vi "Review_Scan_Data.vi"(8 "error in (no error)":errorcluster) -> (0 "error out":errorcluster)   [LabVIEW 2017]
uses:
  Q Driver/Controls/Review_Q options.ctl
  Q Driver/Controls/Review EnQ.ctl
  Controls/Main Cluster.ctl
  Controls/GUI Reference Cluster.ctl
  SQL/SQL/SQL_DB-Enum.ctl
  SQL/Detailed Report _Colums_Informatin.ctl
  <vilib>/addons/database/Auxilliary.llb/DB Tools DataTypes.ctl
  DB Driver/DB Driver Main Options.ctl
  <vilib>/addons/database/NI_Database_API.lvlib
panel:
  out "Machine Tested TIME":dbl(knob) scale=0.0..3000.0
  in  "Search Type":string(combo)="Date&Time"
  out "TESTED":dbl(slide) scale=0.0..10.0
  out "FAIL":dbl(slide) scale=0.0..10.0
  out "PASS":dbl(slide) scale=0.0..10.0
  in  "Table":i32(listbox)=-1
  in  "Password":string caption="User_Name"
  in  "User ID":string caption="User_Name"
  out "DB Name":string
  out "DB Connection Status":string
  out "User Instruction":string
  in  "Export to Pdf":bool
  in  "Close":bool
  in  "Export to CSV":bool
  in  "All/ Top 1000":bool
  in  "Select Field":string(combo)
  in  "Tables":string(combo)
  in  "Field Data":string
  in  "To Date":timestamp
  in  "From Date":timestamp
  in  "Search Data":bool
  out "Connection":bool
  in  "Connect":bool
  out "SERVER NAME :":string
  out "date/time string":string="Wednesday, November 13 2013 2:41:59 PM"
  # "Data Base Connection"
  # "User ID"
  # "Password"
  # "Report Viewer"
  # "Search And Export"
  # "To Date"
  # "From Date"
  # "S.No"
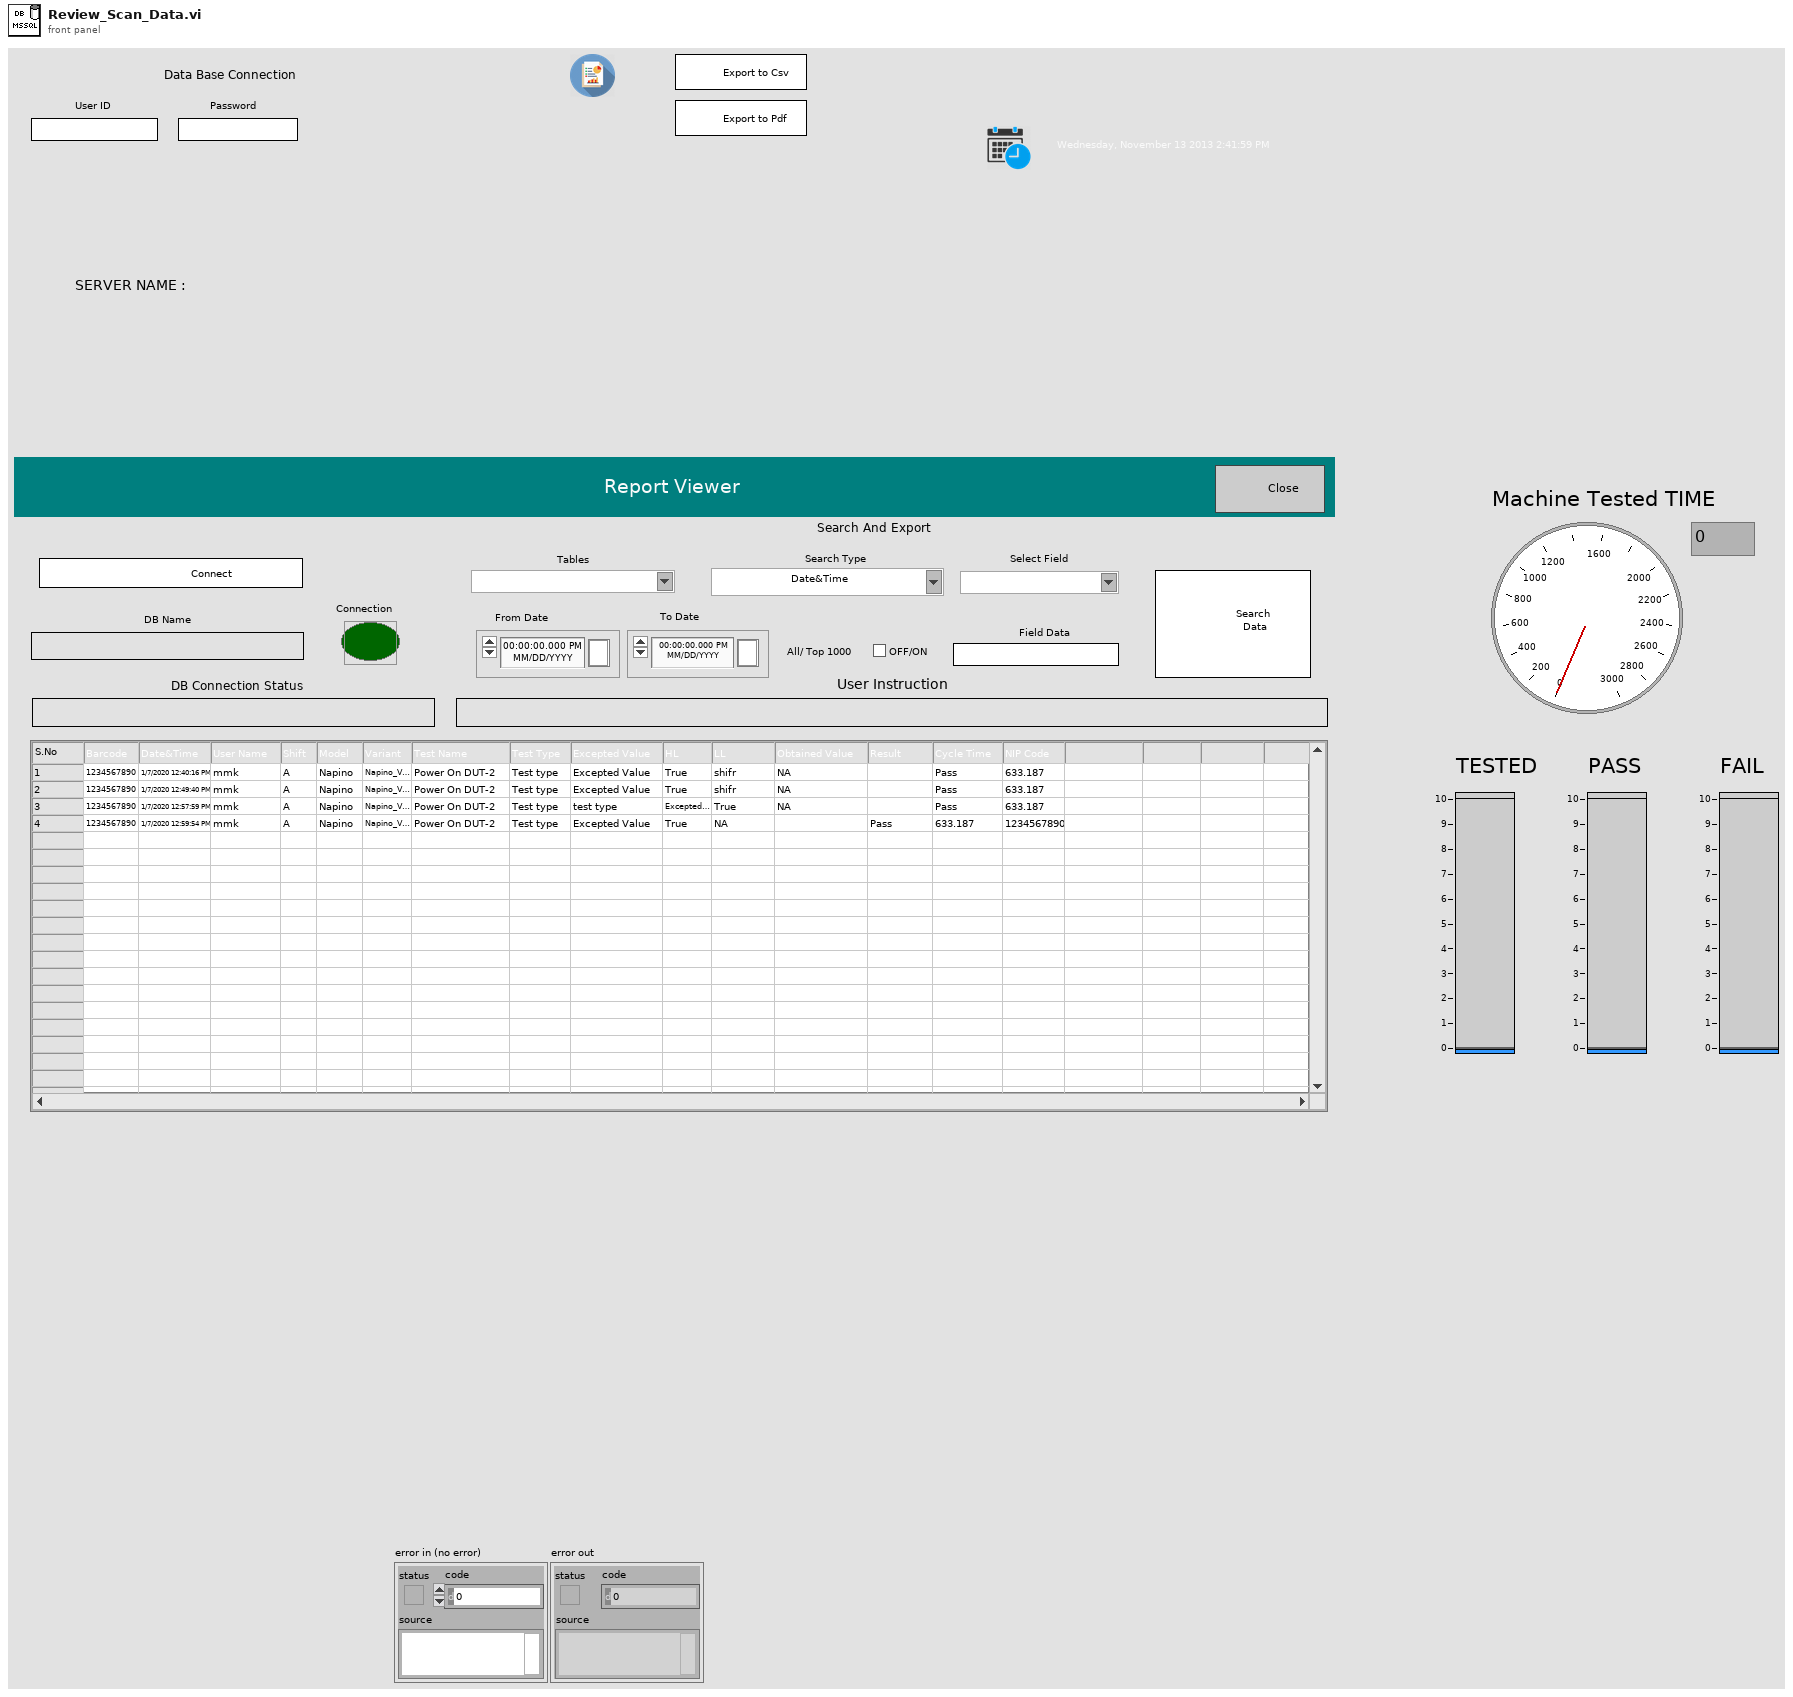
[diagram p1: front panel]
types:
  T1 = typedef "Main Cluster.ctl" = cluster{"From Date":timestamp, "To Date":timestamp, "Selected Database":string, "Selected Table":string, "Selected Field":string, "Field Data":string, "DB Connection Ststus":string, "User Instruction":string, "All/ Top 1000":bool, "Table Data":string[][], "Query":string, "Selected Server":string, "Connection Status":bool, "User ID":string, "Password":string, "Date/Field":bool, "(Date/Field/All)":enum8{"False", "True", "Mixed"}, "First Run":bool, "Selected DB Tables":string[], "From Date Field":string, "To Date Field":string, "Selected Table Fields":string[], "Search Type":string, "Reference":T2, "Mahine RUN Time":dbl, "Pass/Fail querry":string}
  T2 = typedef "GUI Reference Cluster.ctl" = cluster{"Top 1000/ All":refnum<vi>, "Search by date":refnum<vi>, "From Date":refnum<vi>, "Select Field":refnum<vi>, "Field Data":refnum<vi>, "To Date":refnum<vi>, "Tables":refnum<vi>, "Search Type":refnum<vi>}
  T3 = typedef "Review EnQ.ctl" = enum16{"Poll", "Init", "Connect", "Close", "Generate Query", "Update", "Take All Reference", "Check Tables & Create", "Read DB", "Export to Pdf", "Export to Csv", "Error", "Exit"}
  T4 = typedef "Review_Q options.ctl" = enum16{"Init", "En Q", "EN Q N", "EN Q Stack", "EN Q Stack N", "De Q", "Flush", "Close"}
  T5 = typedef "SQL_DB-Enum.ctl" = enum16{"INI DATA", "Open Connections", "Query", "Update Table", "Get Full Report", "Get Serial Numbers", "Get Table Columns", "Get Table Names", "Check & Create Table", "Close Connection"}
  T6 = typedef "Detailed Report _Colums_Informatin.ctl" = cluster{"column name":string, "data type":T7, "size":i32, "allow null?":bool}[]
  T7 = typedef "NI_Database_API.lvlib/DB Tools DataTypes.ctl" = enum16{"String", "Long (I32)", "Single (SGL)", "Double (DBL)", "Date/Time", "Binary"}
  T8 = typedef "DB Driver Main Options.ctl" = enum16{"Open", "RefOut", "Select", "Execute", "Update", "Insert 2D", "Insert OrUpdate", "Close"}
  T9 = cluster{"left":i16, "top":i16, "right":i16, "bottom":i16}
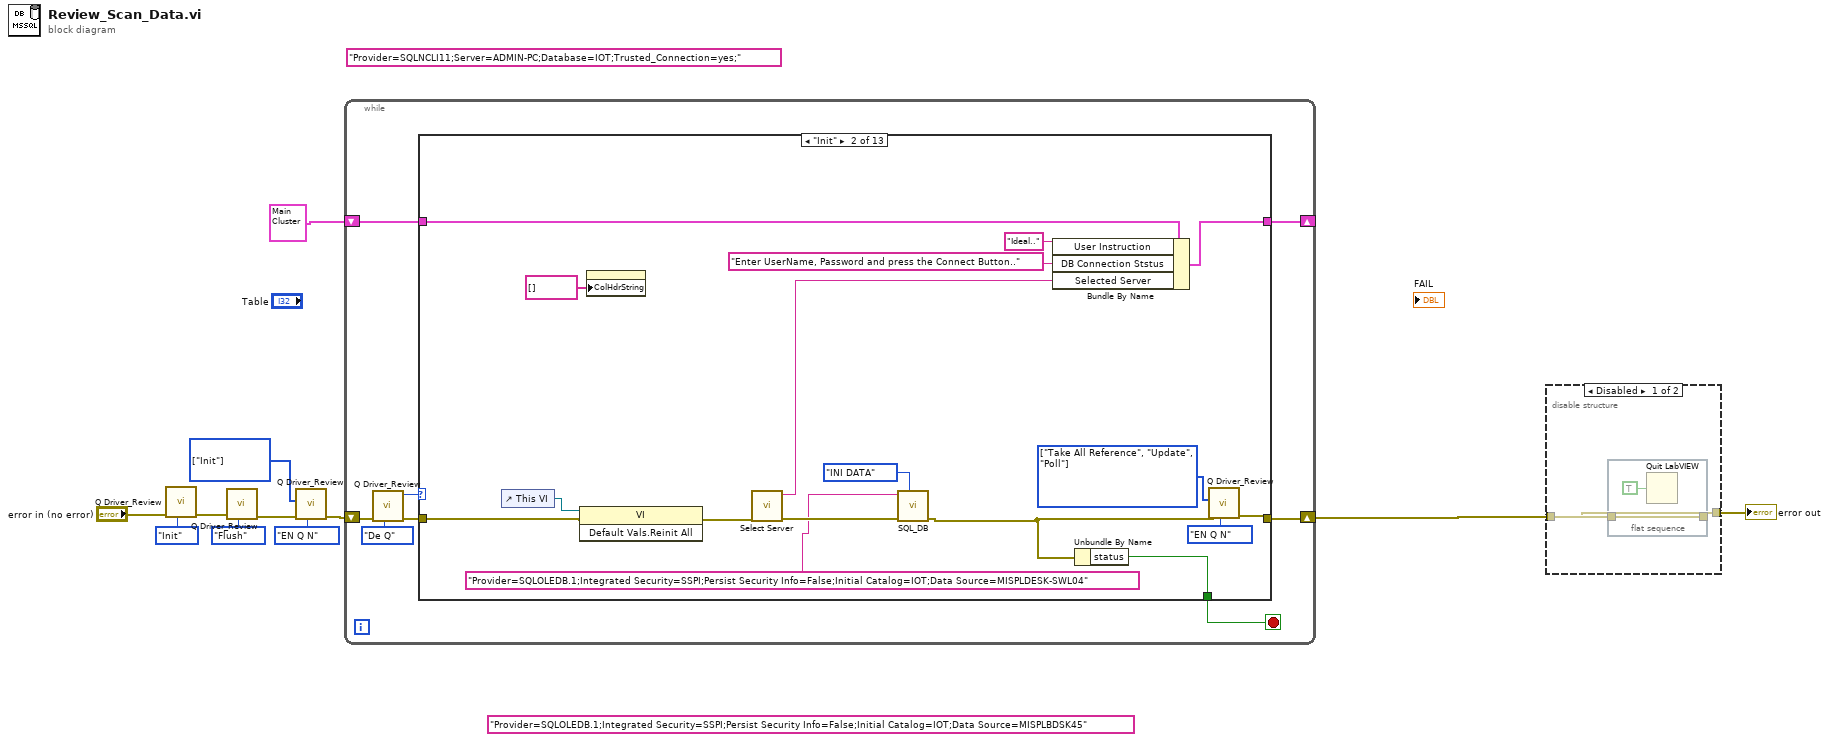
[diagram p0: block diagram]
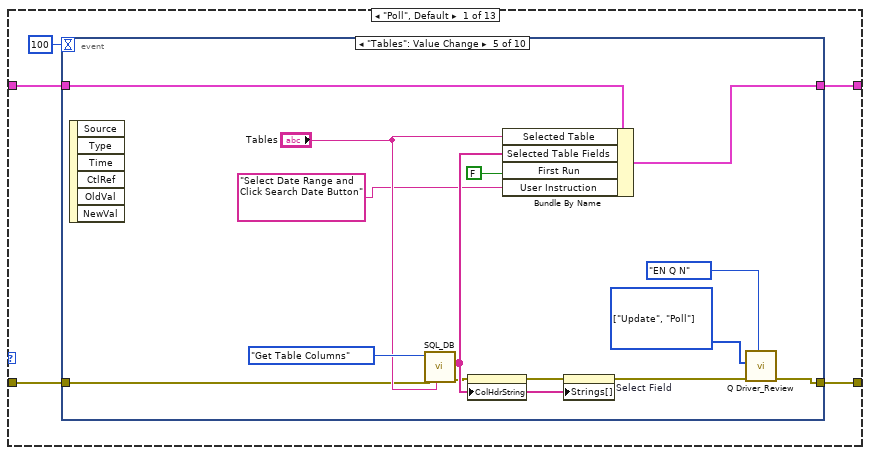
[diagram p3: hidden frame]
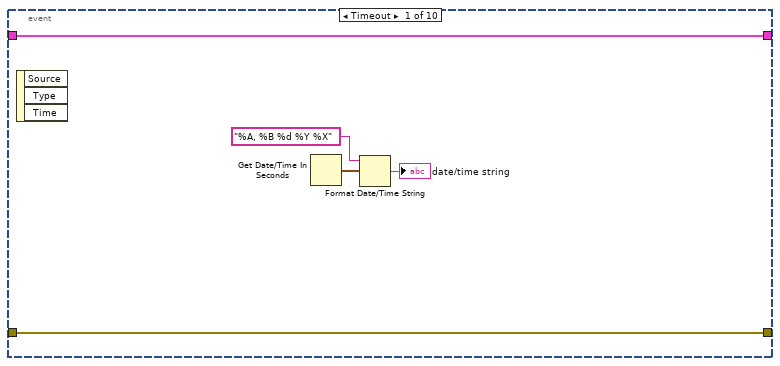
[diagram p4: hidden frame]
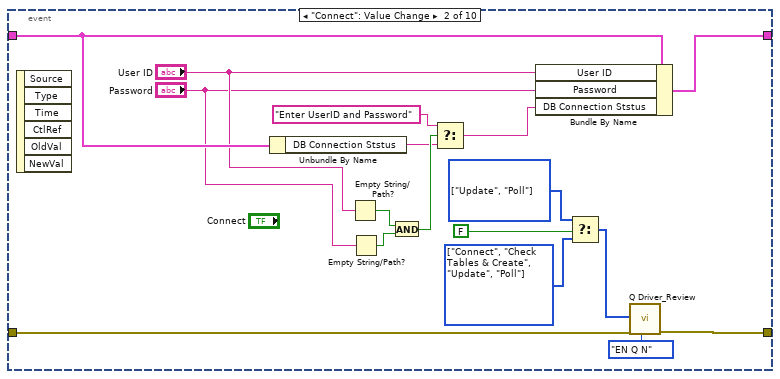
[diagram p5: hidden frame]
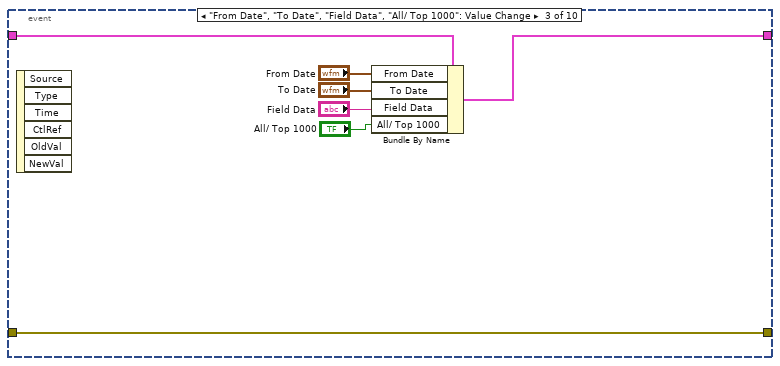
[diagram p6: hidden frame]
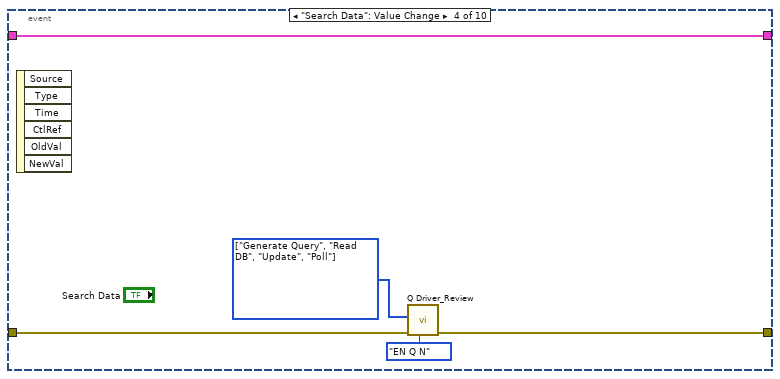
[diagram p7: hidden frame]
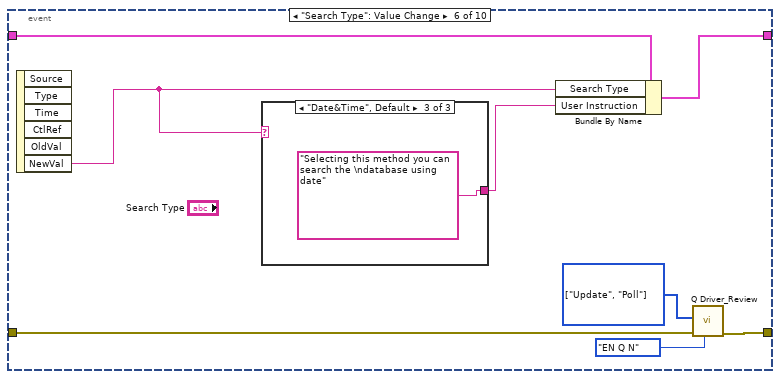
[diagram p8: hidden frame]
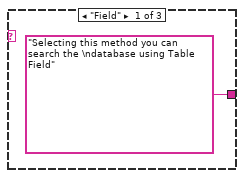
[diagram p9: hidden frame]
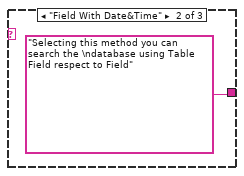
[diagram p10: hidden frame]
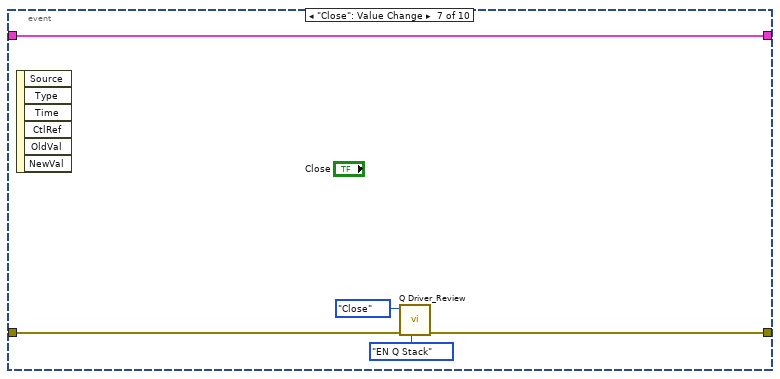
[diagram p11: hidden frame]
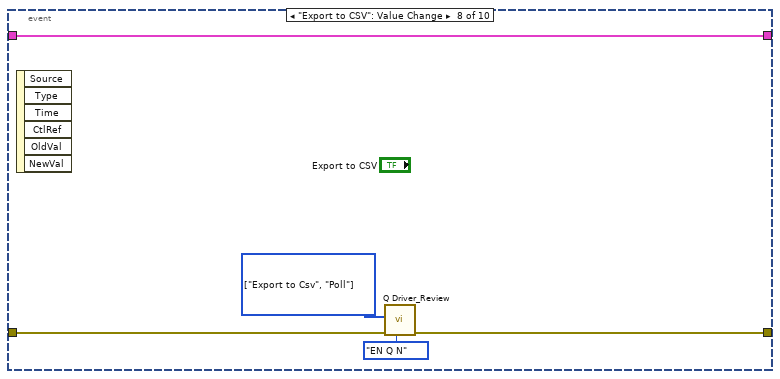
[diagram p12: hidden frame]
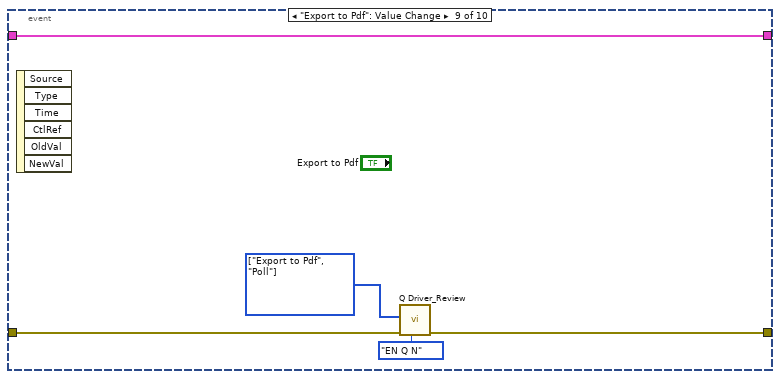
[diagram p13: hidden frame]
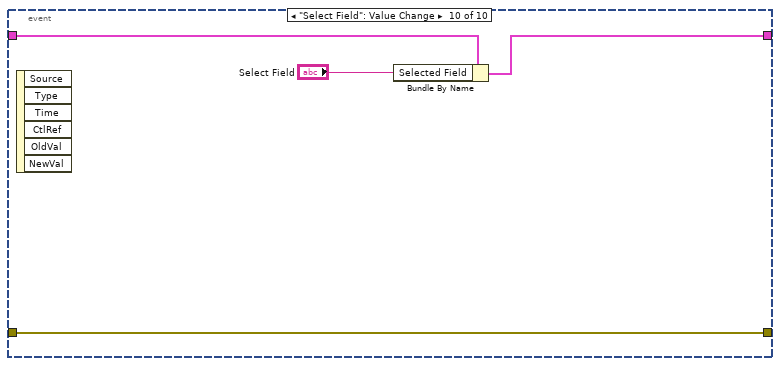
[diagram p14: hidden frame]
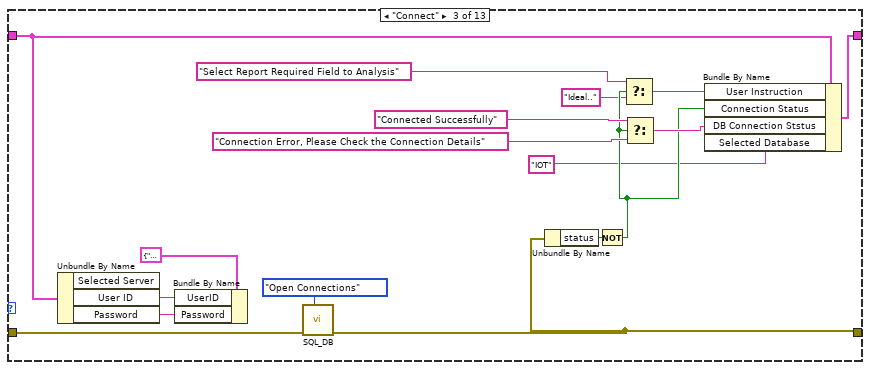
[diagram p15: hidden frame]
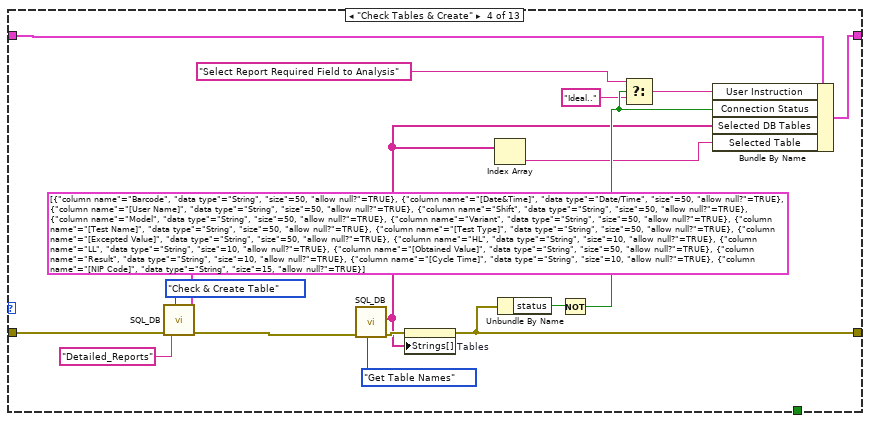
[diagram p16: hidden frame]
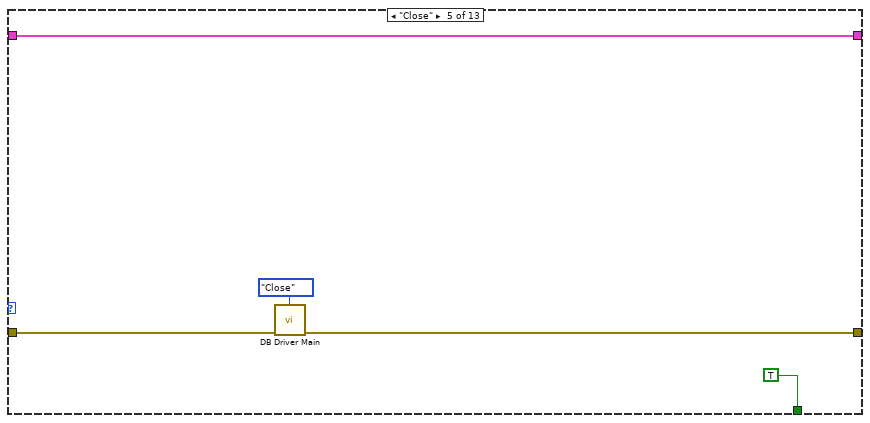
[diagram p17: hidden frame]
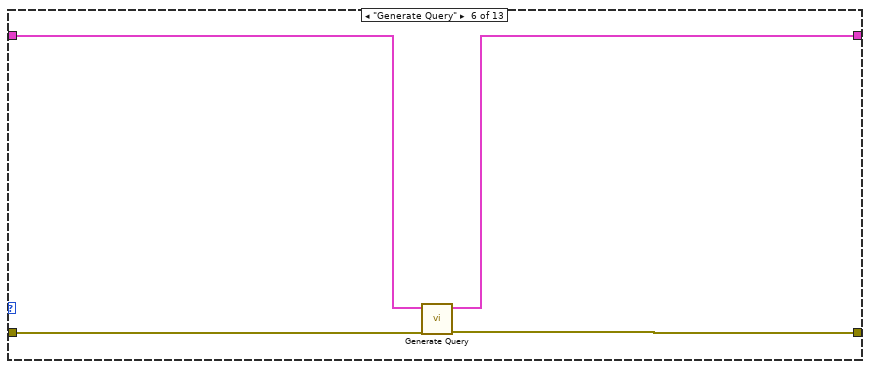
[diagram p18: hidden frame]
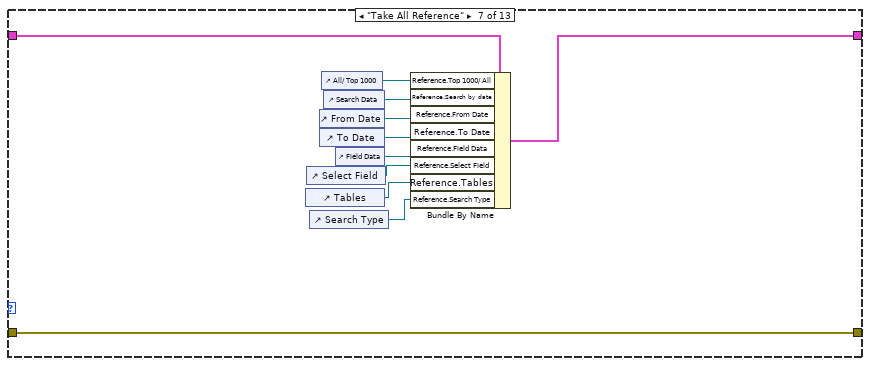
[diagram p19: hidden frame]
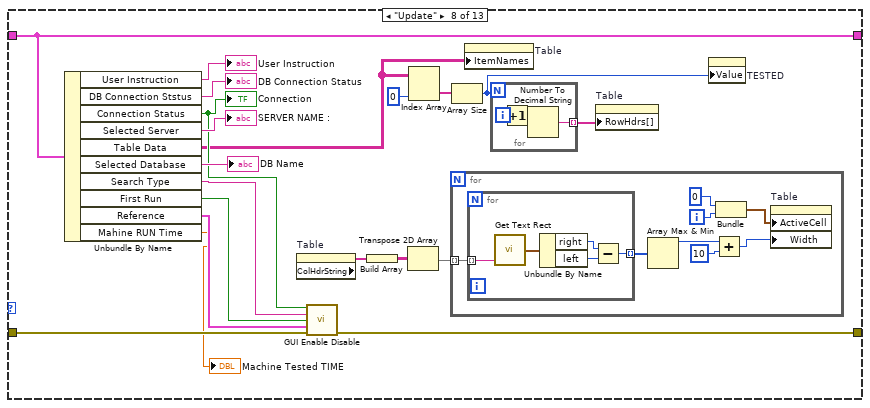
[diagram p20: hidden frame]
diagram:
  (unwired) "Provider=SQLOLEDB.1;Integrated Security=SSPI;Persist Security Info=False;Initial Catalog=IOT;Data Source=MISPLBDSK45" ("Connection Info")
  (unwired) "Provider=SQLNCLI11;Server=ADMIN-PC;Database=IOT;Trusted_Connection=yes;" ("Connection Info")
  w6 = T3[] [enum."Init"] items=["Poll", "Init", "Connect", "Close", "Generate Query", "Update", "Take All Reference", "Check Tables & Create", "Read DB", "Export to Pdf", "Export to Csv", "Error", "Exit"] ("EN Q N")
  n1 = call "Q Driver_Review.vi"("Q Options"=Review_Q_options."Init", "error in (no error)"="error in (no error)") -> ("error out"=w9:errorcluster)  [unwired: 8 in, 1 out]
  n2 = call "Q Driver_Review.vi"("Q Options"=Review_Q_options."Flush", "error in (no error)"=w9) -> ("error out"=w7:errorcluster)  [unwired: 8 in, 1 out]
  n3 = call "Q Driver_Review.vi"("Q Options"=Review_Q_options."EN Q N", "error in (no error)"=w7, "EN Q N"=w6) -> ("error out"=w5:errorcluster)  [unwired: 7 in, 1 out]
  n4 = while {
    shift-right: [w15] -> w2
    shift-left: w5 -> [w18]
    shift-right: [w13] -> _
    shift-left: T1 {"From Date"=timestamp(0 s since 1904-01-01), "To Date"=timestamp(0 s since 1904-01-01), "Selected Database"="", "Selected Table"="", "Selected Field"="", "Field Data"="", "DB Connection Ststus"="", "User Instruction"="", "All/ Top 1000"=FALSE, "Table Data"=[], "Query"="", "Selected Server"="", "Connection Status"=FALSE, "User ID"="", "Password"="", "Date/Field"=FALSE, "(Date/Field/All)"=enum."False", "First Run"=TRUE, "Selected DB Tables"=[], "From Date Field"="", "To Date Field"="", "Selected Table Fields"=[], "Search Type"="", "Reference"={"Top 1000/ All"=refnum, "Search by date"=refnum, "From Date"=refnum, "Select Field"=refnum, "Field Data"=refnum, "To Date"=refnum, "Tables"=refnum, "Search Type"=refnum}, "Mahine RUN Time"=0.0, "Pass/Fail querry"=""} -> [w14]
    stop <- w12 stop-if-true
    n5 = call "Q Driver_Review.vi"("Q Options"=Review_Q_options."De Q", "error in (no error)"=w18) -> ("error out"=w16:errorcluster, "De Q"=w17:T3)  [unwired: 8 in]
    n6 = case shown="\"Init\"" w17 {
      tunnel: w16 -> [w23 w118 w136 w141 w157 w162 w165 w188 w230 w236 w242 w245 w248]
      tunnel: [w22 w110 w121 w142 w154 w161 w165 w182 w217 w235 w241 w244 w247] -> w15
      tunnel: w14 -> [w21 w116 w131 w152 w156 w160 w173 w192 w229 w234 w240 w243 w250]
      tunnel: [w20 w115 w130 w151 w156 w159 w172 w192 w228 w234 w240 w243 w250] -> w13
      tunnel: [_ w104 _ _ TRUE _ _ _ _ _ _ _ TRUE] -> w12
      frame "Poll", Default {
        n7 = event shown="[4] \"Tables\": Value Change" {
          selector: _ -> [_ _ _ _ _ _ _ _ _ _]
          dyn-events: _ -> [_ _ _ _ _ _ _ _ _ _]
          timeout: 100 -> [_ _ _ _ _ _ _ _ _ _]
          tunnel: w23 -> [w26 w44 w49 w56 w67 w77 w86 w91 w96 w99]
          tunnel: [w26 w43 w49 w55 w61 w76 w85 w90 w95 w99] -> w22
          tunnel: w21 -> [w25 w37 w53 w54 w72 w80 w88 w89 w94 w102]
          tunnel: [w25 w46 w52 w54 w71 w79 w88 w89 w94 w100] -> w20
          event Timeout {
            n8 = event-data() -> ()  [unwired: 1 in, 3 out]
            n9 = Get Date/Time In Seconds() -> (seconds since 1Jan1904=w29:timestamp)
            n10 = Format Date/Time String(time format string (%c)="%A, %B %d %Y %X", seconds (now)=w29) -> (date/time string=→"date/time string":string)  [unwired: 1 out]
          }
          event "Connect": Value Change {
            w39 = T3[] [enum."Connect", enum."Check Tables & Create", enum."Update", enum."Poll"] items=["Poll", "Init", "Connect", "Close", "Generate Query", "Update", "Take All Reference", "Check Tables & Create", "Read DB", "Export to Pdf", "Export to Csv", "Error", "Exit"] ("EN Q N")
            w40 = T3[] [enum."Update", enum."Poll"] items=["Poll", "Init", "Connect", "Close", "Generate Query", "Update", "Take All Reference", "Check Tables & Create", "Read DB", "Export to Pdf", "Export to Csv", "Error", "Exit"] ("EN Q N")
            n11 = event-data() -> ()  [unwired: 1 in, 6 out]
            n12 = Unbundle By Name(w37) -> ("DB Connection Ststus"=w35:string)
            n13 = Empty String/Path?(string/path="User ID") -> (empty?=w41:bool)
            n14 = Empty String/Path?(string/path="Password") -> (empty?=w42:bool)
            n15 = And(x=w41, y=w42) -> (x .and. y?=w36:bool)
            n16 = Select(t="Enter UserID and Password", s=w36, f=w35) -> (s? t:f=w33:string)
            n17 = Bundle By Name(cluster=w37, "User ID"="User ID", "Password"="Password", "DB Connection Ststus"=w33) -> (w46:T1)
            n18 = Select(t=w40, s=FALSE, f=w39) -> (s? t:f=w38:T3[])
            n19 = call "Q Driver_Review.vi"("Q Options"=Review_Q_options."EN Q N", "error in (no error)"=w44, "EN Q N"=w38) -> ("error out"=w43:errorcluster)  [unwired: 7 in, 1 out]
          }
          event "From Date", "To Date", "Field Data", "All/ Top 1000": Value Change {
            n20 = event-data() -> ()  [unwired: 1 in, 6 out]
            n21 = Bundle By Name(cluster=w53, "From Date"="From Date", "To Date"="To Date", "Field Data"="Field Data", "All/ Top 1000"="All/ Top 1000") -> (w52:T1)
          }
          event "Search Data": Value Change {
            w57 = T3[] [enum."Generate Query", enum."Read DB", enum."Update", enum."Poll"] items=["Poll", "Init", "Connect", "Close", "Generate Query", "Update", "Take All Reference", "Check Tables & Create", "Read DB", "Export to Pdf", "Export to Csv", "Error", "Exit"] ("EN Q N")
            n22 = event-data() -> ()  [unwired: 1 in, 6 out]
            n23 = call "Q Driver_Review.vi"("Q Options"=Review_Q_options."EN Q N", "error in (no error)"=w56, "EN Q N"=w57) -> ("error out"=w55:errorcluster)  [unwired: 7 in, 1 out]
          }
          event "Tables": Value Change {
            w63 = T3[] [enum."Update", enum."Poll"] items=["Poll", "Init", "Connect", "Close", "Generate Query", "Update", "Take All Reference", "Check Tables & Create", "Read DB", "Export to Pdf", "Export to Csv", "Error", "Exit"] ("EN Q N")
            n24 = event-data() -> ()  [unwired: 1 in, 6 out]
            n25 = call "SQL_DB.vi"("Table Name"="Tables", "CTRL"=SQL_DB-Enum."Get Table Columns", "error in (no error)"=w67) -> ("error in (no error) 2"=w66:errorcluster, "Table/Columns"=w68:string[])  [unwired: 6 in, 1 out]
            n26 = property on="Table" class="MCListbox (strict)"(error in=w66, "ColHdrString"=w68) -> (error out=w65:errorcluster)  [unwired: 1 in, 1 out]
            n27 = Bundle By Name(cluster=w72, "Selected Table"="Tables", "Selected Table Fields"=w68, "First Run"=FALSE, "User Instruction"="Select Date Range and Click Search Date Button") -> (w71:T1)
            n28 = property on="Select Field" class="CmbBox"(error in=w65, "Strings[]"=w68) -> (error out=w62:errorcluster)  [unwired: 1 in, 1 out]
            n29 = call "Q Driver_Review.vi"("Q Options"=Review_Q_options."EN Q N", "error in (no error)"=w62, "EN Q N"=w63) -> ("error out"=w61:errorcluster)  [unwired: 7 in, 1 out]
          }
          event "Search Type": Value Change {
            w75 = T3[] [enum."Update", enum."Poll"] items=["Poll", "Init", "Connect", "Close", "Generate Query", "Update", "Take All Reference", "Check Tables & Create", "Read DB", "Export to Pdf", "Export to Csv", "Error", "Exit"] ("EN Q N")
            n30 = event-data() -> ("NewVal"=w73:string)  [unwired: 1 in, 5 out]
            n31 = case shown="\"Date&Time\", Default" w73 {
              tunnel: ["Selecting this method you can search the \ndatabase using Table Field" "Selecting this method you can search the \ndatabase using Table Field respect to Field" "Selecting this method you can search the \ndatabase using date"] -> w74
              frame "Field" {
              }
              frame "Field With Date&Time" {
              }
              frame "Date&Time", Default {
              }
            }
            n32 = Bundle By Name(cluster=w80, "Search Type"=w73, "User Instruction"=w74) -> (w79:T1)
            n33 = call "Q Driver_Review.vi"("Q Options"=Review_Q_options."EN Q N", "error in (no error)"=w77, "EN Q N"=w75) -> ("error out"=w76:errorcluster)  [unwired: 7 in, 1 out]
          }
          event "Close": Value Change {
            n34 = event-data() -> ()  [unwired: 1 in, 6 out]
            n35 = call "Q Driver_Review.vi"("Q Options"=Review_Q_options."EN Q Stack", "error in (no error)"=w86, "En Q"=Review_EnQ."Close") -> ("error out"=w85:errorcluster)  [unwired: 7 in, 1 out]
          }
          event "Export to CSV": Value Change {
            w92 = T3[] [enum."Export to Csv", enum."Poll"] items=["Poll", "Init", "Connect", "Close", "Generate Query", "Update", "Take All Reference", "Check Tables & Create", "Read DB", "Export to Pdf", "Export to Csv", "Error", "Exit"] ("EN Q N")
            n36 = event-data() -> ()  [unwired: 1 in, 6 out]
            n37 = call "Q Driver_Review.vi"("Q Options"=Review_Q_options."EN Q N", "error in (no error)"=w91, "EN Q N"=w92) -> ("error out"=w90:errorcluster)  [unwired: 7 in, 1 out]
          }
          event "Export to Pdf": Value Change {
            w97 = T3[] [enum."Export to Pdf", enum."Poll"] items=["Poll", "Init", "Connect", "Close", "Generate Query", "Update", "Take All Reference", "Check Tables & Create", "Read DB", "Export to Pdf", "Export to Csv", "Error", "Exit"] ("EN Q N")
            n38 = event-data() -> ()  [unwired: 1 in, 6 out]
            n39 = call "Q Driver_Review.vi"("Q Options"=Review_Q_options."EN Q N", "error in (no error)"=w96, "EN Q N"=w97) -> ("error out"=w95:errorcluster)  [unwired: 7 in, 1 out]
          }
          event "Select Field": Value Change {
            n40 = event-data() -> ()  [unwired: 1 in, 6 out]
            n41 = Bundle By Name(cluster=w102, "Selected Field"="Select Field") -> (w100:T1)
          }
        }
      }
      frame "Init" {
        w111 = T3[] [enum."Take All Reference", enum."Update", enum."Poll"] items=["Poll", "Init", "Connect", "Close", "Generate Query", "Update", "Take All Reference", "Check Tables & Create", "Read DB", "Export to Pdf", "Export to Csv", "Error", "Exit"] ("EN Q N")
        n42 = control-ref of="This VI"() -> (w119:refnum<vi>)
        n43 = invoke class="VI" method="Default Vals.Reinit All"(reference=w119, error in=w118) -> (error out=w117:errorcluster)  [unwired: 1 in, 2 out]
        n44 = property on="Table" class="MCListbox (strict)"("ColHdrString"=string[] [] ("Column Header Strings[]")) -> ()  [unwired: 2 in, 2 out]
        n45 = call "Select Server.vi"("error in (no error)"=w117) -> ("error out"=w107:errorcluster, "Selected Database"=w114:string)  [unwired: 9 in]
        n46 = call "SQL_DB.vi"("CTRL"=SQL_DB-Enum."INI DATA", "error in (no error)"=w107, "Connection Info"="Provider=SQLOLEDB.1;Integrated Security=SSPI;Persist Security Info=False;Initial Catalog=IOT;Data Source=MISPLDESK-SWL04") -> ("error in (no error) 2"=w106:errorcluster)  [unwired: 6 in, 2 out]
        n47 = Bundle By Name(cluster=w116, "User Instruction"="Ideal..", "DB Connection Ststus"="Enter UserName, Password and press the Connect Button..", "Selected Server"=w114) -> (w115:T1)
        n48 = Unbundle By Name(w106) -> ("status"=w104:bool)
        n49 = call "Q Driver_Review.vi"("Q Options"=Review_Q_options."EN Q N", "error in (no error)"=w106, "EN Q N"=w111) -> ("error out"=w110:errorcluster)  [unwired: 7 in, 1 out]
      }
      frame "Connect" {
        n50 = Unbundle By Name(w131) -> ("User ID"=w134:string, "Password"=w133:string)  [unwired: 1 out]
        n51 = Bundle By Name(cluster=cluster{"UserID":string, "Password":string} {"UserID"="sa", "Password"="12345"} ("DB Connection Details"), "UserID"=w134, "Password"=w133) -> ()  [unwired: 1 out]
        n52 = call "SQL_DB.vi"("CTRL"=SQL_DB-Enum."Open Connections", "error in (no error)"=w136) -> ("error in (no error) 2"=w121:errorcluster)  [unwired: 7 in, 2 out]
        n53 = Unbundle By Name(w121) -> ("status"=w132:bool)
        n54 = Not(x=w132) -> (.not. x?=w126:bool)
        n55 = Select(t="Select Report Required Field to Analysis", s=w126, f="Ideal.." ("User Instruction")) -> (s? t:f=w123:string)
        n56 = Select(t="Connected Successfully", s=w126, f="Connection Error, Please Check the Connection Details") -> (s? t:f=w127:string)
        n57 = Bundle By Name(cluster=w131, "User Instruction"=w123, "Connection Status"=w126, "DB Connection Ststus"=w127, "Selected Database"="IOT" ("Table /DBName/Query")) -> (w130:T1)
      }
      frame "Check Tables & Create" {
        n58 = call "SQL_DB.vi"("column information"=T6 [{"column name"="Barcode", "data type"=enum."String", "size"=50, "allow null?"=TRUE}, {"column name"="[Date&Time]", "data type"=enum."Date/Time", "size"=50, "allow null?"=TRUE}, {"column name"="[User Name]", "data type"=enum."String", "size"=50, "allow null?"=TRUE}, {"column name"="Shift", "data type"=enum."String", "size"=50, "allow null?"=TRUE}, {"column name"="Model", "data type"=enum."String", "size"=50, "allow null?"=TRUE}, {"column name"="Variant", "data type"=enum."String", "size"=50, "allow null?"=TRUE}, {"column name"="[Test Name]", "data type"=enum."String", "size"=50, "allow null?"=TRUE}, {"column name"="[Test Type]", "data type"=enum."String", "size"=50, "allow null?"=TRUE}, {"column name"="[Excepted Value]", "data type"=enum."String", "size"=50, "allow null?"=TRUE}, {"column name"="HL", "data type"=enum."String", "size"=10, "allow null?"=TRUE}, {"column name"="LL", "data type"=enum."String", "size"=10, "allow null?"=TRUE}, {"column name"="[Obtained Value]", "data type"=enum."String", "size"=50, "allow null?"=TRUE}, {"column name"="Result", "data type"=enum."String", "size"=10, "allow null?"=TRUE}, {"column name"="[Cycle Time]", "data type"=enum."String", "size"=10, "allow null?"=TRUE}, {"column name"="[NIP Code]", "data type"=enum."String", "size"=15, "allow null?"=TRUE}] ("Array 2"), "Table Name"="Detailed_Reports" ("table"), "CTRL"=SQL_DB-Enum."Check & Create Table", "error in (no error)"=w141) -> ("error in (no error) 2"=w138:errorcluster)  [unwired: 5 in, 2 out]
        n59 = call "SQL_DB.vi"("CTRL"=SQL_DB-Enum."Get Table Names", "error in (no error)"=w138) -> ("error in (no error) 2"=w145:errorcluster, "Table/Columns"=w144:string[])  [unwired: 7 in, 1 out]
        n60 = property on="Tables" class="CmbBox"(error in=w145, "Strings[]"=w144) -> (error out=w142:errorcluster)  [unwired: 1 in, 1 out]
        n61 = Index Array(array=w144) -> (element=w143:string)  [unwired: 1 in]
        n62 = Unbundle By Name(w142) -> ("status"=w153:bool)
        n63 = Not(x=w153) -> (.not. x?=w150:bool)
        n64 = Select(t="Select Report Required Field to Analysis", s=w150, f="Ideal.." ("User Instruction")) -> (s? t:f=w147:string)
        n65 = Bundle By Name(cluster=w152, "User Instruction"=w147, "Connection Status"=w150, "Selected DB Tables"=w144, "Selected Table"=w143) -> (w151:T1)
      }
      frame "Close" {
        n66 = call "DB Driver Main.vi"("Option"=DB_Driver_Main_Options."Close", "error in"=w157) -> ("error out"=w154:errorcluster)  [unwired: 9 in, 4 out]
      }
      frame "Generate Query" {
        n67 = call "Generate Query.vi"("error in (no error)"=w162, "Cluster In"=w160) -> ("error out"=w161:errorcluster, "Cluster Out"=w159:T1)  [unwired: 8 in]
      }
      frame "Take All Reference" {
        n68 = control-ref of="Tables"() -> (w164:refnum<vi>)
        n69 = control-ref of="Select Field"() -> (w166:refnum<vi>)
        n70 = control-ref of="Search Type"() -> (w163:refnum<vi>)
        n71 = control-ref of="From Date"() -> (w169:refnum<vi>)
        n72 = control-ref of="To Date"() -> (w168:refnum<vi>)
        n73 = control-ref of="All/ Top 1000"() -> (w171:refnum<vi>)
        n74 = control-ref of="Search Data"() -> (w170:refnum<vi>)
        n75 = control-ref of="Field Data"() -> (w167:refnum<vi>)
        n76 = Bundle By Name(cluster=w173, "Reference.Top 1000/ All"=w171, "Reference.Search by date"=w170, "Reference.From Date"=w169, "Reference.To Date"=w168, "Reference.Field Data"=w167, "Reference.Select Field"=w166, "Reference.Tables"=w164, "Reference.Search Type"=w163) -> (w172:T1)
      }
      frame "Update" {
        n77 = Unbundle By Name(w192) -> ("User Instruction"=→"User Instruction":string, "DB Connection Ststus"=→"DB Connection Status":string, "Connection Status"=w186:bool, "Selected Server"=→"SERVER NAME :":string, "Table Data"=w181:string[][], "Selected Database"=→"DB Name":string, "Search Type"=w175:string, "First Run"=w187:bool, "Reference"=w185:T2, "Mahine RUN Time"=→"Machine Tested TIME":dbl)
        "Connection" <- w186
        n78 = property on="Table" class="MCListbox (strict)"() -> ("ColHdrString"=w178:string[])  [unwired: 2 in, 2 out]
        n79 = call "GUI Enable Disable.vi"("Connection Ststus"=w186, "Search Type"=w175, "First Run"=w187, "Reference"=w185, "error in (no error)"=w188) -> ("error out"=w182:errorcluster)  [unwired: 10 in]
        n80 = Build Array(w178) -> (w180:string[][])
        n81 = Transpose 2D Array(2D array=w180) -> (transposed array=w179:string[][])
        n82 = Index Array(array=w181, index (col)=0 ("disabled index (col)")) -> (element=w177:string[])  [unwired: 1 in]
        n83 = for {
          tunnel: w179 -> [w201] mode=indexing
          i -> [w197]
          n84 = for {
            tunnel: w201 -> [w206] mode=indexing
            tunnel: [w202] -> w200 mode=indexing
            n85 = call <vilib>:"Get Text Rect.vi"("text"=w206) -> ("rect"=w205:T9)  [unwired: 8 in]
            n86 = Unbundle By Name(w205) -> ("right"=w204:i16, "left"=w203:i16)
            n87 = Subtract(x=w204, y=w203) -> (x-y=w202:i16)
          }
          n88 = Array Max & Min(array=w200) -> (max value=w196:i16)  [unwired: 3 out]
          n89 = Add(x=w196, y=i16 10) -> (x+y=w194:i16)
          n90 = Bundle(0, w197) -> (w195:cluster{i32, i32})  [unwired: 1 in]
          n91 = property on="Table" class="MCListbox (strict)"("ActiveCell"=w195, "Width"=w194) -> ()  [unwired: 2 in, 2 out]
        }
        n92 = Array Size(array=w177) -> (size(s)=w176:i32)
        n93 = property on="Table" class="MCListbox (strict)"("ItemNames"=w181) -> ()  [unwired: 2 in, 2 out]
        n94 = for {
          N: w176 -> [_]
          tunnel: [w208] -> w184 mode=indexing
          i -> [w209]
          n95 = Increment(x=w209) -> (x+1=w207:i32)
          n96 = Number To Decimal String(number=w207) -> (decimal integer string=w208:string)  [unwired: 1 in]
        }
        n97 = property on="Table" class="MCListbox (strict)"("RowHdrs[]"=w184) -> ()  [unwired: 2 in, 2 out]
        n98 = property on="TESTED" class="Slide (strict)"("Value"=w176) -> ()  [unwired: 2 in, 2 out]
      }
      frame "Read DB" {
        w219 = SQL_DB-Enum."Get Full Report" ("CTRL")
        n99 = Unbundle By Name(w229) -> ("Pass/Fail querry"=w216:string, "Query"=w231:string)
        n100 = call "SQL_DB.vi"("CTRL"=w219, "error in (no error)"=w230, "SQL query"=w231) -> ("error in (no error) 2"=w218:errorcluster, "Data out 2"=w215:string[][])  [unwired: 6 in, 1 out]
        n101 = call "SQL_DB.vi"("CTRL"=w219, "error in (no error)"=w218, "SQL query"=w216) -> ("error in (no error) 2"=w217:errorcluster, "Data out 2"=w212:string[][])  [unwired: 6 in, 1 out]
        n102 = Array Size(array=w212) -> (size(s)=w211:i32[])
        n103 = Index Array(array=w215, index (col)=13 ("disabled index (col)")) -> (element=w222:string[])  [unwired: 1 in]
        n104 = Array Size(array=w215) -> (size(s)=w214:i32[])
        n105 = Fract/Exp String To Number(string=w222) -> (number=w221:dbl[])  [unwired: 3 in, 1 out]
        n106 = Empty Array?(array=w215) -> (empty?=w227:bool)
        n107 = Add Array Elements(numeric array=w221) -> (sum=w220:dbl)
        n108 = Index Array(array=w211) -> (element=→"PASS":i32)  [unwired: 1 in]
        n109 = Index Array(array=w214) -> (element=→"TESTED":i32)  [unwired: 1 in]
        n110 = Select(t="No Data available for this selection..", s=w227, f="Press Export button to get the report as Pdf or Csv file format") -> (s? t:f=w224:string)
        n111 = Bundle By Name(cluster=w229, "User Instruction"=w224, "Table Data"=w215, "Mahine RUN Time"=w220) -> (w228:T1)
      }
      frame "Export to Pdf" {
        n112 = property on="Table" class="MCListbox (strict)"() -> ("ColHdrString"=w233:string[], "ItemNames"=w232:string[][])  [unwired: 2 in, 2 out]
        n113 = call "Report Driver.vi"("error in"=w236, "2D Data"=w232, "Header Data"=w233) -> ("error out"=w235:errorcluster)  [unwired: 7 in, 1 out]
      }
      frame "Export to Csv" {
        n114 = property on="Table" class="MCListbox (strict)"() -> ("ColHdrString"=w239:string[], "ItemNames"=w238:string[][])  [unwired: 2 in, 2 out]
        n115 = Build Array (concatenate)(w239, w238) -> (w237:string[][])
        n116 = call "Export to csv.vi"("error in (no error)"=w242, "Table Data"=w237) -> ("error out"=w241:errorcluster)  [unwired: 9 in]
      }
      frame "Error" {
        n117 = call <vilib>:"Clear Errors.vi"("error in (no error)"=w245) -> ("error out"=w244:errorcluster)  [unwired: 5 in, 1 out]
      }
      frame "Exit" {
        n118 = call "SQL_DB.vi"("CTRL"=SQL_DB-Enum."Close Connection", "error in (no error)"=w248) -> ("error in (no error) 2"=w247:errorcluster)  [unwired: 7 in, 2 out]
      }
    }
  }
  n119 = disable-structure shown="Disabled" {
    disable-tunnel: w2 -> [w252 _]
    disable-tunnel: [w251 _] -> w1
    frame Disabled {
      n120 = flat-sequence {
        tunnel: w252 -> [w253]
        tunnel: [w253] -> w251
        frame #0 {
          n121 = Quit LabVIEW(quit? (T)=TRUE) -> ()
        }
      }
    }
    frame Enabled {
    }
  }
  "error out" <- w1
